vi "Execute Delete Caption.vi"(6 "Mouse Position":T1, 8 "User VI Ref":refnum<vi>, 9 "Menu Item Tag Suffix":string, 10 "Remaining Items":refnum<vi>[](array[refnum]), 11 "Affected Items":cluster{"Controls":refnum<vi>[]}) -> (0 "Fail transaction?":bool)   [LabVIEW 2020]
doc: "This VI is part of a plug-in for modifying the LabVIEW shortcut menus. This is the execute VI which is called when the shortcut menu is chosen by the user. It performs the action of the selected menu item."
uses:
  <vilib>/Utility/miscctls.llb/LVPositionTypeDef.ctl
panel:
  # "All controls on this panel except \"Affected Items\" have been locked to prevent accidental edits. Changing the control names or types, other than the elements of the \"Affected Items\" cluster will make the VI unusable as a menu plugin.\n\nSee Context Help for each control for details about its use."
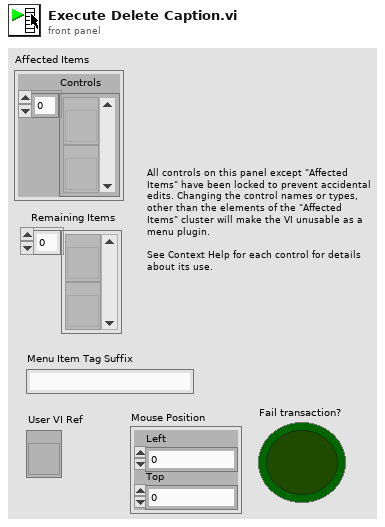
[diagram p1: front panel]
types:
  T1 = typedef "LVPositionTypeDef.ctl" = cluster{"Left":i32, "Top":i32}
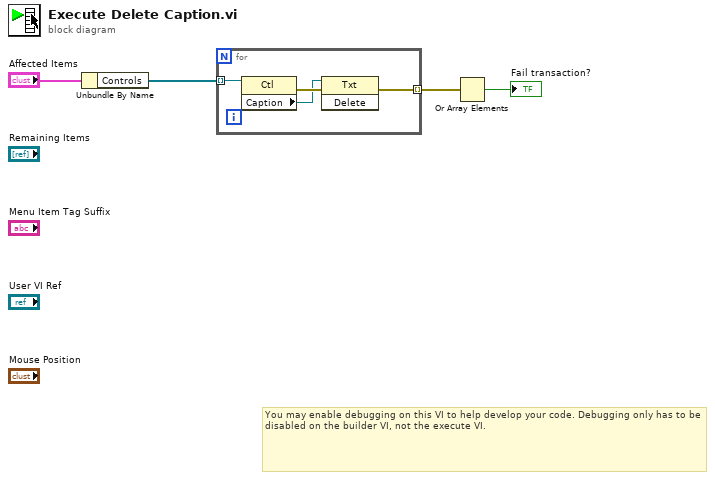
[diagram p0: block diagram]
diagram:
  # "You may enable debugging on this VI to help develop your code. Debugging only has to be disabled on the builder VI, not the execute VI."
  n1 = Unbundle By Name("Affected Items") -> ("Controls"=w3:refnum<vi>[])
  n2 = for {
    tunnel: w3 -> [w7] mode=indexing
    tunnel: [w5] -> w2 mode=indexing
    n3 = property class="Ctl"(reference=w7) -> (error out=w8:errorcluster, "Caption"=w6:refnum<vi>)  [unwired: 1 in, 1 out]
    n4 = invoke class="Txt" method="Delete"(reference=w6, error in=w8) -> (error out=w5:errorcluster)  [unwired: 1 in, 2 out]
  }
  n5 = Or Array Elements(Boolean array=w2) -> (logical OR=→"Fail transaction?":bool)
